vi "PXIe-433x Timing Source.vi"(8 "error in (no error)":errorcluster, 10 "Loop Time (usec)":u32, 11 "Device Ref":T1=18446744073709551615 format="%.0x") -> (0 "error out":errorcluster, 1 "Primary Control Loop dt":i64, 2 "Actual Loop Rate (Hz)":dbl, 3 "Timing Source Name":string)   [LabVIEW 2011, in "PXIe-433x Custom Device.lvlib"]
uses:
  PXIe-433x Custom Device.lvlib
  <vilib>/NI Veristand/Custom Device API/Custom Device Item Ref.ctl
  Global.vi
  <vilib>/NI Veristand/Custom Device API/Get Item Property (Boolean).vi
  <vilib>/NI Veristand/Custom Device Tools/Custom Device Utility Library/NI VeriStand - Search for All Items by GUID.vi
  <vilib>/DAQmx/configure/timing.llb/DAQmx Timing (Sample Clock).vi
  <vilib>/DAQmx/configure/events/hardwareSignals.llb/DAQmx Export Signal (Most Signals).vi
  <vilib>/DAQmx/create/timing.llb/DAQmx Create Timing Source (Signal From Task).vi
  <vilib>/NI Veristand/Custom Device Tools/Custom Device Utility Library/Custom Device Utility Library.lvlib
  <vilib>/NI Veristand/Custom Device API/Custom Device API.lvlib
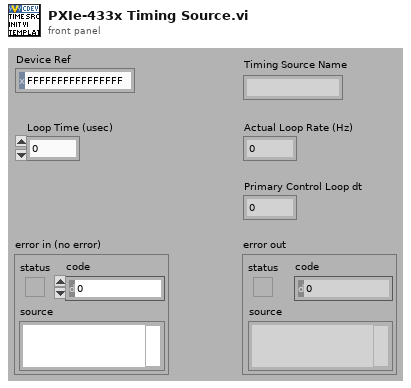
[diagram p1: front panel]
types:
  T1 = typedef "Custom Device API.lvlib/Custom Device Item Ref.ctl" = u64
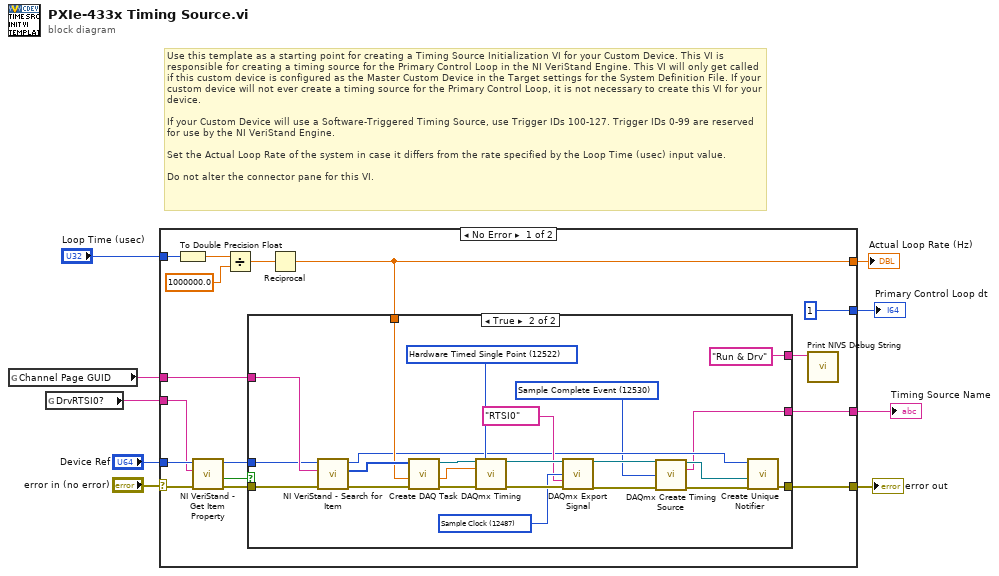
[diagram p0: block diagram]
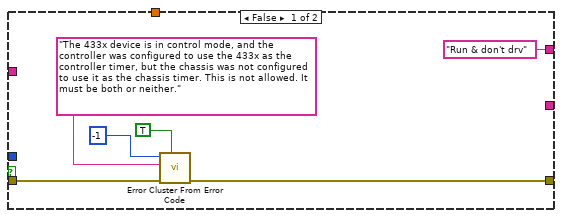
[diagram p2: hidden frame]
diagram:
  # "Use this template as a starting point for creating a Timing Source Initialization VI for your Custom Device. This VI is responsible for creating a timing source for the Primary Control Loop in the NI VeriStand Engine. This VI will only get called if this custom device is configured as the Master Custom Device in the Target settings for the System Definition File. If your custom device will not ever create a timing source for the Primary Control Loop, it is not necessary to create this VI for your device.\n\nIf your Custom Device will use a Software-Triggered Timing Source, use Trigger IDs 100-127. Trigger IDs 0-99 are reserved for use by the NI VeriStand Engine.\n\nSet the Actual Loop Rate of the system in case it differs from the rate specified by the Loop Time (usec) input value.\n\nDo not alter the connector pane for this VI."
  n1 = global read "Global.vi" "Channel Page GUID"() -> (w4:string)
  n2 = global read "Global.vi" "DrvRTSI0?"() -> (w2:string)
  n3 = case shown="No Error" "error in (no error)" {
    selector: "error in (no error)" -> [w18 w55]
    tunnel: [w12 w55] -> w9
    tunnel: "Loop Time (usec)" -> [w25 _]
    tunnel: [w21 _] -> w6
    tunnel: "Device Ref" -> [w17 _]
    tunnel: w4 -> [w20 _]
    tunnel: [i64 1 ("Primary Control Loop dt") _] -> w3
    tunnel: w2 -> [w16 _]
    tunnel: [w11 _] -> w1
    frame No Error {
      n4 = To Double Precision Float(number=w25) -> (double precision float=w24:dbl)
      n5 = call-poly <vilib>:"NI VeriStand - Get Item Property.vi"("error in (no error)"=w18, "Property Name"=w16, "Item Ref in"=w17) -> ("error out"=w14:errorcluster, "Value"=w13:bool, "Item Ref out"=w15:T1)  [unwired: 5 in, 1 out]
      n6 = Divide(x=w24, y=1000000.0) -> (x/y=w22:dbl)
      n7 = Reciprocal(x=w22) -> (1/x=w21:dbl)
      n8 = case shown="True" w13 {
        tunnel: w21 -> [_ w52]
        tunnel: w20 -> [_ w51]
        tunnel: w15 -> [_ w50]
        tunnel: w14 -> [w28 w49]
        tunnel: [w27 w40] -> w12
        tunnel: [_ w34] -> w11
        tunnel: ["Run & don't drv" "Run & Drv"] -> w10
        frame False {
          n9 = call <vilib>:"Error Cluster From Error Code.vi"("show call chain? (False)"=TRUE, "error in (no error)"=w28, "error message (\"\")"="The 433x device is in control mode, and the controller was configured to use the 433x as the controller timer, but the chassis was not configured to use it as the chassis timer. This is not allowed. It must be both or neither." ("error message (\"\")"), "error code (0)"=-1) -> ("error out"=w27:errorcluster)  [unwired: 5 in]
        }
        frame True {
          w32 = 12530 items=["Sample Complete Event"=12530, "Counter Output Event"=12494, "Change Detection Event"=12511, "Sample Clock"=12487] ("signal")
          w42 = 12487 items=["AI Convert Clock"=12484, "10MHz Reference Clock"=12536, "20MHz Timebase Clock"=12486, "Sample Clock"=12487, "Advance Trigger"=12488, "Reference Trigger"=12490, "Start Trigger"=12491, "Advance Complete Event"=12492, "AI Hold Complete Event"=12493, "Counter Output Event"=12494, "Change Detection Event"=12511, "Watchdog Timer Expired Event"=12512] ("signal")
          w47 = 12522 items=["Finite Samples"=10178, "Continuous Samples"=10123, "Hardware Timed Single Point"=12522] ("sample mode")
          n10 = call-poly <vilib>:"NI VeriStand - Search for Item.vi"("error in"=w49, "Item GUID"=w51, "Section Ref in"=w50) -> ("error out"=w54:errorcluster, "Item Refs"=w53:T1[], "Section Ref out"=w35:T1)  [unwired: 5 in, 1 out]
          n11 = call "Create DAQ Task.vi"("error in"=w54, "User provided rate"=w52, "Channels"=w53) -> ("error out"=w46:errorcluster, "Actual rate"=w45:dbl, "task out"=w48:refnum<k21>)  [unwired: 6 in]
          n12 = call-poly <vilib>:"DAQmx Timing.vi"("task/channels in"=w48, "sample mode"=w47, "rate"=w45, "error in"=w46) -> ("task out"=w44:refnum<k21>, "error out"=w43:errorcluster)  [unwired: 10 in]
          n13 = call-poly <vilib>:"DAQmx Export Signal.vi"("task/channels in"=w44, "signal"=w42, "output terminal"=tag "RTSI0", "error in"=w43) -> ("task out"=w38:refnum<k21>, "error out"=w39:errorcluster)  [unwired: 10 in]
          n14 = call-poly <vilib>:"DAQmx Create Timing Source.vi"("task/channels in"=w38, "signal"=w32, "error in"=w39) -> ("task out"=w36:refnum<k21>, "timing source out"=w34:string, "error out"=w37:errorcluster)  [unwired: 10 in]
          n15 = call "Create Unique Notifier.vi"("error in"=w37, "DAQ task to send"=w36, "Device Ref"=w35) -> ("error out"=w40:errorcluster)  [unwired: 5 in, 3 out]
        }
      }
      n16 = call "Print NIVS Debug String.vi"("Debug String"=w10) -> ()  [unwired: 9 in, 1 out]
    }
    frame Error {
    }
  }
  "error out" <- w9
  "Timing Source Name" <- w1
  "Actual Loop Rate (Hz)" <- w6
  "Primary Control Loop dt" <- w3
